vi "EditGraph.vi"(8 "Error":errorcluster, 9 "Graph Index":i32, 10 "Tag":string, 11 "Tree in":refnum<class "Tree.lvclass">) -> (0 "Error":errorcluster, 1 "Selected Element":T1, 2 "Found?":bool, 3 "Tree out":refnum<class "Tree.lvclass">)   [LabVIEW 2021, in "Tree.lvlib" / "Tree.lvclass"]
uses:
  Tree.lvclass
  Private/TreeControllerTag.ctl
  Tree.lvclass/Tree.ctl
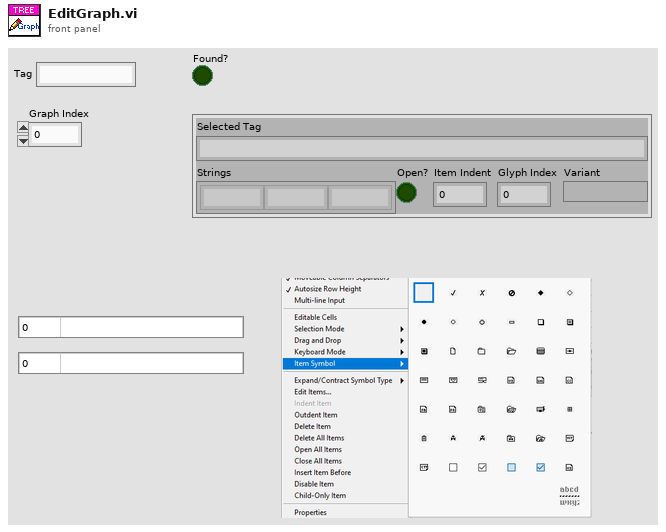
[diagram p1: front panel]
types:
  T1 = cluster{"Selected Tag":string, "Strings":string[], "Open?":bool, "Item Indent":i32, "Glyph Index":i32, "Variant":variant}
  T2 = cluster{"Found":bool, "Selected Element":cluster{"Selected Tag":string, "Strings":string[], "Open?":bool, "Item Indent":i32, "Glyph Index":i32, "Variant":variant}}
  T3 = cluster{enum16{"EditStrings", "EditGraph", "EditVariant"}, "Tag":string, "Value":variant}
  T4 = enum16{"EditStrings", "EditGraph", "EditVariant"}
  T5 = typedef "Tree.lvlib/Tree.lvclass/TreeControllerTag.ctl" = enum8{"Null", "1. Add item", "2. Delete item", "3. Get All Tree Data", "4. Drag Starting", "5. Drag Ended", "6. Add Tree Values", "7. Get Item Value", "8. Edit Item", "9. StepBack", "10. Filter"}
  T6 = cluster{"cluster":cluster{enum16{"EditStrings", "EditGraph", "EditVariant"}, "Tag":string, "Value":variant}, "queue out":refnum<queue>}
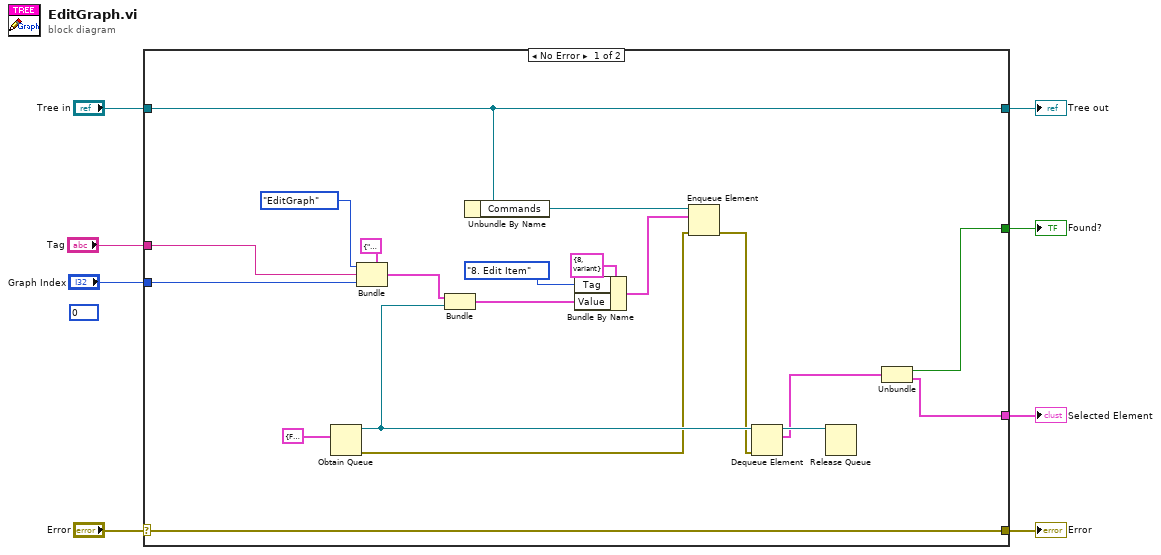
[diagram p0: block diagram]
diagram:
  (unwired) 0
  n1 = case shown="No Error" "Error" {
    selector: "Error" -> [w28 w30]
    tunnel: [w28 w30] -> w7
    tunnel: [w27 w29] -> w5
    tunnel: "Tree in" -> [w27 w29]
    tunnel: "Graph Index" -> [w9 _]
    tunnel: [w15 _] -> w3
    tunnel: "Tag" -> [w19 _]
    tunnel: [w14 _] -> w1
    frame No Error {
      n2 = Obtain Queue(element data type=T2 {"Found"=FALSE, "Selected Element"={"Selected Tag"="", "Strings"=[], "Open?"=FALSE, "Item Indent"=0, "Glyph Index"=0, "Variant"=variant}} ("output cluster")) -> (queue out=w22:refnum<queue>, error out=w12:errorcluster)  [unwired: 4 in, 1 out]
      n3 = Bundle(cluster=T3 {enum."EditStrings", "Tag"="", "Value"=variant}, T4."EditGraph", "Tag"=w19, "Value"=w9) -> (w20:T3)
      n4 = Bundle("cluster"=w20, "queue out"=w22) -> (w23:T6)  [unwired: 1 in]
      n5 = Unbundle By Name(w27) -> ("Commands"=w26:refnum<queue>)
      n6 = Bundle By Name(cluster=cluster{"Tag":u8, "Value":variant} {"Tag"=8, "Value"=variant} ("element"), "Tag"=TreeControllerTag."8. Edit Item", "Value"=w23) -> (w24:cluster{"Tag":u8, "Value":variant})
      n7 = Enqueue Element(queue=w26, element=w24, error in (no error)=w12) -> (error out=w13:errorcluster)  [unwired: 1 in, 2 out]
      n8 = Dequeue Element(queue=w22, error in (no error)=w13) -> (queue out=w21:refnum<queue>, element=w16:T2)  [unwired: 1 in, 2 out]
      n9 = Release Queue(queue=w21) -> ()  [unwired: 2 in, 3 out]
      n10 = Unbundle(w16) -> ("Found"=w15:bool, "Selected Element"=w14:T1)
    }
    frame Error {
    }
  }
  "Error" <- w7
  "Tree out" <- w5
  "Found?" <- w3
  "Selected Element" <- w1
